vi "Configure Offset and Limits (Spectrum Emission Mask - VBW).vi"(0 "VISA resource name":refnum<visa-resource-name>, 1 "Auto VBW/RBW Ratio":bool[](array[boolean])=[FALSE, FALSE, FALSE, FALSE, FALSE, FALSE], 2 "Manual VBW/RBW Ratio":dbl[](array[numeric])=[0.01, 0.01, 0.01, 0.01, 0.01, 0.01] format="%#.6g", 5 "Device Mode (1: BTS)":i32(ring)=1 items=["BTS"=1, "MS"=2], 11 "error in (no error)":errorcluster, 12 "Auto Video Bandwidth List":bool[](array[boolean])=[FALSE, FALSE, FALSE, FALSE, FALSE, FALSE], 13 "Manual Video Bandwidth List":dbl[](array[numeric])=[300.0, 300.0, 300.0, 300.0, 300.0, 300.0] format="%#.6g") -> (4 "VISA resource name out":refnum<visa-resource-name>, 15 "error out":errorcluster)   [LabVIEW 2018, in "Agilent MXA Series.lvlib"]
doc: "Configures the VBW settings under the offsets and limits for Spectrum Emission Mask measurement type."
uses:
  Agilent MXA Series.lvlib
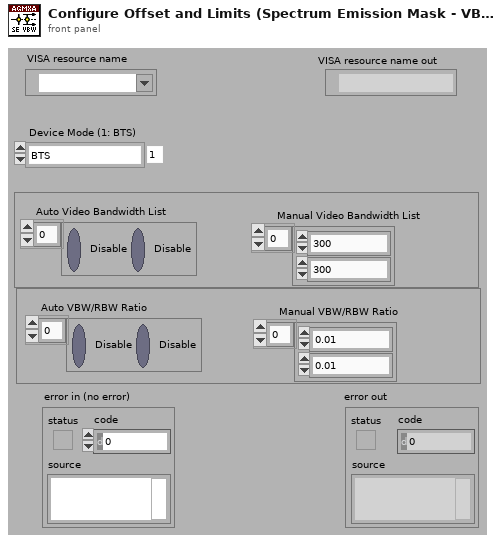
[diagram p1: front panel]
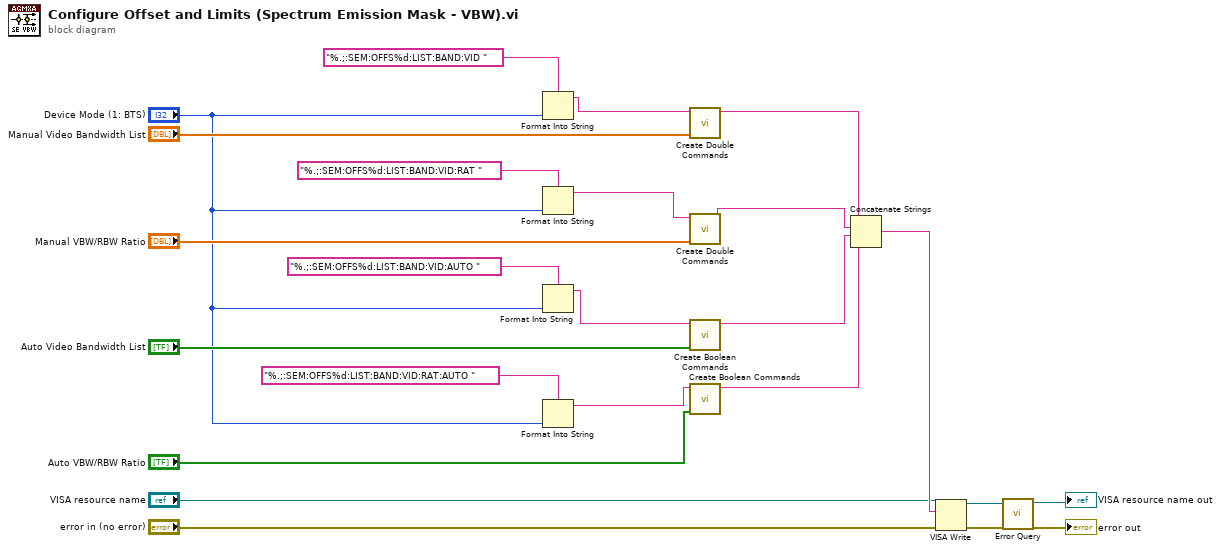
[diagram p0: block diagram]
diagram:
  n1 = Format Into String(format string="%.;:SEM:OFFS%d:LIST:BAND:VID " ("initial string"), "Device Mode (1: BTS)") -> (resulting string=w23:string)  [unwired: 2 in, 1 out]
  n2 = Format Into String(format string="%.;:SEM:OFFS%d:LIST:BAND:VID:RAT " ("initial string"), "Device Mode (1: BTS)") -> (resulting string=w20:string)  [unwired: 2 in, 1 out]
  n3 = Format Into String(format string="%.;:SEM:OFFS%d:LIST:BAND:VID:AUTO " ("initial string"), "Device Mode (1: BTS)") -> (resulting string=w17:string)  [unwired: 2 in, 1 out]
  n4 = Format Into String(format string="%.;:SEM:OFFS%d:LIST:BAND:VID:RAT:AUTO " ("initial string"), "Device Mode (1: BTS)") -> (resulting string=w13:string)  [unwired: 2 in, 1 out]
  n5 = call "Create Double Commands.vi"("Double Values"="Manual Video Bandwidth List", "Commands"=w23) -> ("Result"=w11:string)  [unwired: 9 in]
  n6 = call "Create Double Commands.vi"("Double Values"="Manual VBW/RBW Ratio", "Commands"=w20) -> ("Result"=w10:string)  [unwired: 9 in]
  n7 = call "Create Boolean Commands.vi"("Boolean States"="Auto Video Bandwidth List", "Command"=w17) -> ("Result String"=w9:string)  [unwired: 9 in]
  n8 = call "Create Boolean Commands.vi"("Boolean States"="Auto VBW/RBW Ratio", "Command"=w13) -> ("Result String"=w8:string)  [unwired: 9 in]
  n9 = Concatenate Strings(w11, w10, w9, w8) -> (w5:string)
  n10 = VISA Write(VISA resource name="VISA resource name", write buffer=w5, error in (no error)="error in (no error)") -> (VISA resource name out=w6:refnum<visa-resource-name>, error out=w7:errorcluster)  [unwired: 1 out]
  n11 = call "Error Query.vi"("error in (no error)"=w7, "VISA resource name"=w6) -> ("error out"=→"error out":errorcluster, "VISA resource name out"=→"VISA resource name out":refnum<visa-resource-name>)  [unwired: 6 in, 2 out]
